vi "main.vi"() -> ()   [LabVIEW 2011]
uses:
  Controls/Full_90 Degree Pulse Settings.ctl
  Controls/90D_Delay Settings.ctl
  Controls/90D_Preliminary Settings.ctl
  Controls/90D_Pulse Settings.ctl
  Controls/Acquisition Settings.ctl
  Controls/Full_CPMG Degree Pulse Settings.ctl
  Controls/CPMG_Delay Settings.ctl
  Controls/CPMG_Preliminary Settings.ctl
  Controls/CPMG_Pulse Settings.ctl
  Controls/Full_T1 Degree Pulse Settings.ctl
  Controls/T1_Preliminary Settings.ctl
  Controls/T1_Pulse Settings.ctl
  Controls/T1_Delay Settings.ctl
  Controls/Hardware Control.ctl
  Controls/NMR Pulse Sequence Type.ctl
  Controls/Class Objects.ctl
  Modules/File/Configuration/Configuration.lvclass
  Modules/File/TDMS/TDMS.lvclass
  Modules/Hardware/Power Supply/Power Supply.lvclass
  Modules/Hardware/NMR/NMR.lvclass
  Controls/User Event Control.ctl
  Controls/User Event Action.ctl
  Controls/User Interface Control.ctl
  Controls/User Interface Action.ctl
  <vilib>/Utility/error.llb/DialogType.ctl
  Error Handling/Custom Errors.ctl
  Functional Globals/Pulse Parameters.ctl
  Error Handling/Error Module Action.ctl
  Functional Globals/General Flags.ctl
  Functional Globals/Hardware Parameters.ctl
  Controls/Class Labels.ctl
panel:
  in  "Tab Control":T1(tab)
  out "FFT Graph":cluster{"magnitude":dbl[], dbl[]}[](graph)
  out "Time Graph":cluster{"magnitude":dbl[], dbl[]}[](graph)
  in  "Hardware CTRL":T2={"Number Samples"=5000, "Time Between Points"=10.0, "Gain2 (dB)"=12, "CuttOff Freq1[MHz]"=10, "CuttOff Freq2[MHz]"=1, "Frequency"=10000000.0, "Phase"=180, "Power Level"=230, "Send Pulse"=FALSE, "Reset DDS"=FALSE, "TX CTRL"=FALSE, "RX CTRL"=TRUE, "Gain1 (dB)"=5, "Set DDS"=FALSE, "Start AQS"=FALSE, "Units"=0} {"Units" items=["us", "ms"]; "Gain1 (dB)" min=-5 max=45 step=1; "Power Level" max=1023 step=1; "Phase" max=270 step=90; "Frequency" min=1.0 format="%^#_6e"; "CuttOff Freq2[MHz]" min=1 max=30 step=1; "CuttOff Freq1[MHz]" min=1 max=30 step=1; "Gain2 (dB)" min=-5 max=45 step=1; "Time Between Points" min=0.0 step=1.0; "Number Samples" step=1}
  in  "Save to file":bool
  in  "Sum?":bool=TRUE
  out "Transfer Time (ms)":u32=322
  in  "start sequence  loop":bool
  out "Real (time Domain)":cluster{"magnitude":dbl[], dbl[]}(graph)
  out "Imag (Freq Domain)":cluster{"magnitude":dbl[], dbl[]}(graph)
  in  "Pulse Sequence Type":T3
  in  "90 Degree Pulse Sequence":T4={"Delay Settings"={"Delay d1"=99.98328812669524, "Delay d2"=3.0280548223167, "d1 Unit"=0, "d2 Unit"=1}, "Preliminary Settings"={"Nº of Scans (ns)"=20, "Pulse Frequency"=10000000.0}, "Pulse Settings"={"Duration Signal P1"=20.01128707673462, "Power Level"=800, "Phase"=90, "P1 Units"=0}, "Acquisition Settings"={"Number Samples"=8000, "Time Between Points"=0.0, "Unit"=0}} {"Acquisition Settings"."Unit" items=["us", "ms"]; "Acquisition Settings"."Time Between Points" min=0.0 step=1.0; "Acquisition Settings"."Number Samples" step=1; "Pulse Settings"."P1 Units" items=["us", "ms"]; "Pulse Settings"."Phase" max=270 step=90; "Pulse Settings"."Power Level" max=1023 step=1; "Pulse Settings"."Duration Signal P1" min=0.0 step=1.0 format="%#_4g"; "Preliminary Settings"."Pulse Frequency" min=1.0 max=200000000.0 step=1000000.0 format="%^#_6e"; "Preliminary Settings"."Nº of Scans (ns)" step=1; "Delay Settings"."d2 Unit" items=["us", "ms"]; "Delay Settings"."d1 Unit" items=["us", "ms"]; "Delay Settings"."Delay d2" min=0.0 step=1.0 format="%#_4g"; "Delay Settings"."Delay d1" min=0.0 step=1.0 format="%#_4g"}
  in  "start sequence":bool
  in  "CPMG Pulse Sequence":T9={"Acquisition Settings"={"Number Samples"=500, "Time Between Points"=20.0, "Unit"=0}, "Delay Settings"={"Delay d1"=100.0, "Delay d2"=2.0, "d1 Unit"=0, "d2 Unit"=0, "Delay d3"=100.0, "d3 Unit"=0, "Delay d4"=2.0, "d4 Unit"=0}, "Preliminary Settings"={"Nº of Scans (ns)"=2, "Pulse Frequency"=9000000.0, "Nº of Echoes (ne)"=3}, "Pulse Settings"={"Duration Signal P1"=100.0, "Power Level P1"=1000, "Phase P1"=90, "P1 Unit"=0, "Duration Signal P2"=100.0, "Power Level P2"=1000, "Phase P2"=90, "P2 Unit"=0}} {"Pulse Settings"."P2 Unit" items=["us", "ms"]; "Pulse Settings"."Phase P2" max=270 step=90; "Pulse Settings"."Power Level P2" max=1023 step=1; "Pulse Settings"."Duration Signal P2" min=0.0 step=1.0 format="%#_4g"; "Pulse Settings"."P1 Unit" items=["us", "ms"]; "Pulse Settings"."Phase P1" max=270 step=90; "Pulse Settings"."Power Level P1" max=1023 step=1; "Pulse Settings"."Duration Signal P1" min=0.0 step=1.0 format="%#_4g"; "Preliminary Settings"."Nº of Echoes (ne)" step=1; "Preliminary Settings"."Pulse Frequency" min=1.0 max=200000000.0 step=1000000.0 format="%^#_6e"; "Preliminary Settings"."Nº of Scans (ns)" step=1; "Delay Settings"."d4 Unit" items=["us", "ms"]; "Delay Settings"."Delay d4" min=0.0 step=1.0 format="%#_4g"; "Delay Settings"."d3 Unit" items=["us", "ms"]; "Delay Settings"."Delay d3" min=0.0 step=1.0 format="%#_4g"; "Delay Settings"."d2 Unit" items=["us", "ms"]; "Delay Settings"."d1 Unit" items=["us", "ms"]; "Delay Settings"."Delay d2" min=0.0 step=1.0 format="%#_4g"; "Delay Settings"."Delay d1" min=0.0 step=1.0 format="%#_4g"; "Acquisition Settings"."Unit" items=["us", "ms"]; "Acquisition Settings"."Time Between Points" min=0.0 step=1.0; "Acquisition Settings"."Number Samples" step=1}
  in  "T1 Pulse Sequence":T13={"Preliminary Settings"={"Nº of Scans (ns)"=2, "Pulse Frequency"=9000000.0, "Nº of Vd"=3}, "Pulse Settings"={"Duration Signal P2"=100.0, "Power Level P2"=1000, "Phase P2"=90, "P2 Unit"=0, "Duration Signal P1"=100.0, "Power Level P1"=1000, "Phase P1"=90, "P1 Unit"=0}, "Acquisition Settings"={"Number Samples"=5000, "Time Between Points"=20.0, "Unit"=0}, "Delay Settings"={"Delay d1"=100.0, "Delay d2"=2.0, "d1 Unit"=0, "d2 Unit"=0, "Delay d30"=0.0, "d30 Unit"=0, "Vd Unit"=0, "Vd Values"="Automatic"}} {"Delay Settings"."Vd Unit" items=["us", "ms"]; "Delay Settings"."d30 Unit" items=["us", "ms"]; "Delay Settings"."Delay d30" min=0.0 step=1.0; "Delay Settings"."d2 Unit" items=["us", "ms"]; "Delay Settings"."d1 Unit" items=["us", "ms"]; "Delay Settings"."Delay d2" min=0.0 step=1.0 format="%#_4g"; "Delay Settings"."Delay d1" min=0.0 step=1.0 format="%#_4g"; "Acquisition Settings"."Unit" items=["us", "ms"]; "Acquisition Settings"."Time Between Points" min=0.0 step=1.0; "Acquisition Settings"."Number Samples" step=1; "Pulse Settings"."P1 Unit" items=["us", "ms"]; "Pulse Settings"."Phase P1" max=270 step=90; "Pulse Settings"."Power Level P1" max=1023 step=1; "Pulse Settings"."Duration Signal P1" min=0.0 step=1.0 format="%#_4g"; "Pulse Settings"."P2 Unit" items=["us", "ms"]; "Pulse Settings"."Phase P2" max=270 step=90; "Pulse Settings"."Power Level P2" max=1023 step=1; "Pulse Settings"."Duration Signal P2" min=0.0 step=1.0 format="%#_4g"; "Preliminary Settings"."Nº of Vd" step=1; "Preliminary Settings"."Pulse Frequency" min=1.0 max=200000000.0 step=1000000.0 format="%^#_6e"; "Preliminary Settings"."Nº of Scans (ns)" step=1}
  out "Real (Freq Domain)":cluster{"magnitude":dbl[], dbl[]}(graph)
  out "Imag (time Domain)":cluster{"magnitude":dbl[], dbl[]}(graph)
  out "Sequence Progress":u32(slide)=20 scale=0.0..50.0
  out "Status Bar":string="Sequence Started"
  # "Sequence parameters:\n\nd30 - does not need to be configured"
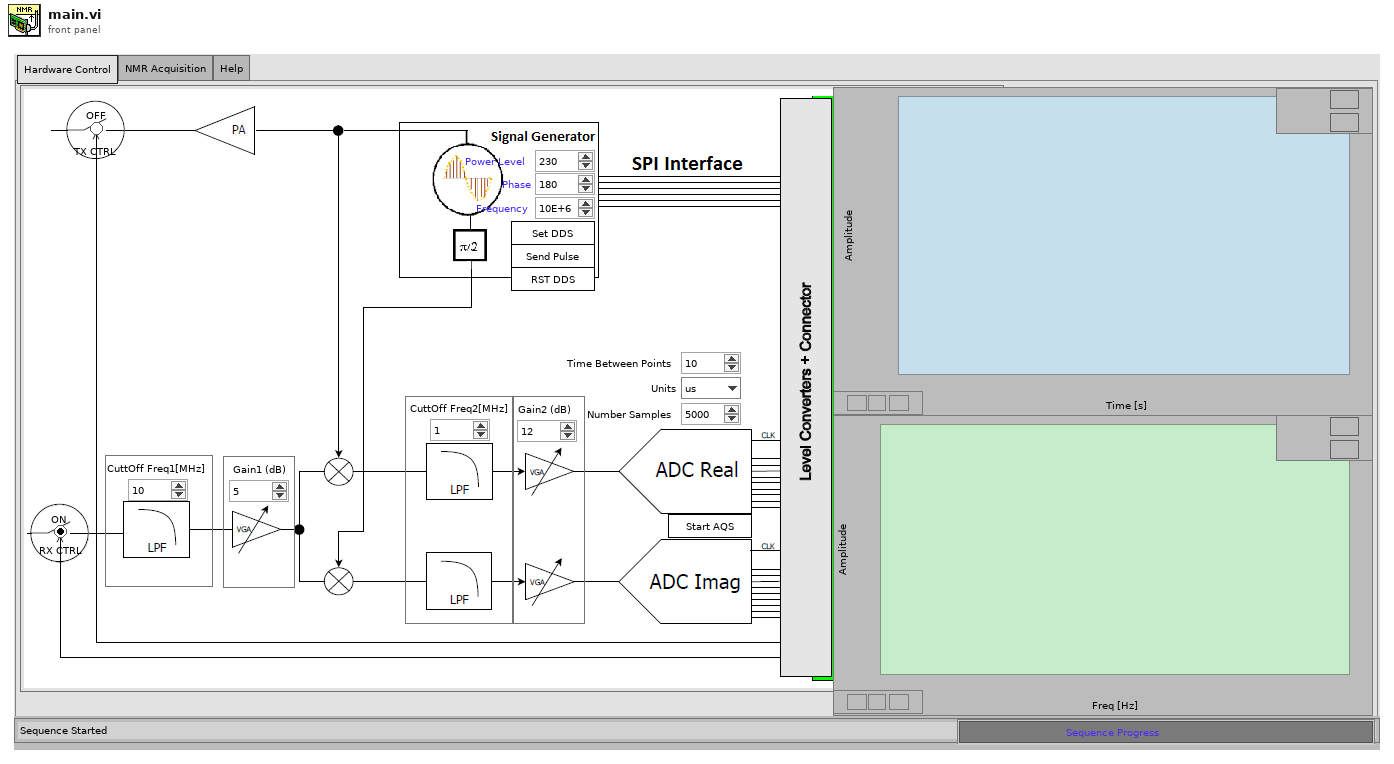
[diagram p1: front panel]
types:
  T1 = enum32{"Hardware Control", "NMR Acquisition", "Help"}
  T2 = typedef "Hardware Control.ctl" = cluster{"Number Samples":u16, "Time Between Points":dbl, "Gain2 (dB)":i8, "CuttOff Freq1[MHz]":u8, "CuttOff Freq2[MHz]":u8, "Frequency":dbl, "Phase":u16, "Power Level":u16, "Send Pulse":bool, "Reset DDS":bool, "TX CTRL":bool, "RX CTRL":bool, "Gain1 (dB)":i8, "Set DDS":bool, "Start AQS":bool, "Units":u8}
  T3 = typedef "NMR Pulse Sequence Type.ctl" = enum16{"90 Degree Sequence", "CPMG Pulse Sequence", "T1 Pulse Sequence"}
  T4 = typedef "Full_90 Degree Pulse Settings.ctl" = cluster{"Delay Settings":T5, "Preliminary Settings":T6, "Pulse Settings":T7, "Acquisition Settings":T8}
  T5 = typedef "90D_Delay Settings.ctl" = cluster{"Delay d1":dbl, "Delay d2":dbl, "d1 Unit":u8, "d2 Unit":u8}
  T6 = typedef "90D_Preliminary Settings.ctl" = cluster{"Nº of Scans (ns)":u16, "Pulse Frequency":dbl}
  T7 = typedef "90D_Pulse Settings.ctl" = cluster{"Duration Signal P1":dbl, "Power Level":u16, "Phase":u16, "P1 Units":u8}
  T8 = typedef "Acquisition Settings.ctl" = cluster{"Number Samples":u16, "Time Between Points":dbl, "Unit":u8}
  T9 = typedef "Full_CPMG Degree Pulse Settings.ctl" = cluster{"Acquisition Settings":T8, "Delay Settings":T10, "Preliminary Settings":T11, "Pulse Settings":T12}
  T10 = typedef "CPMG_Delay Settings.ctl" = cluster{"Delay d1":dbl, "Delay d2":dbl, "d1 Unit":u8, "d2 Unit":u8, "Delay d3":dbl, "d3 Unit":u8, "Delay d4":dbl, "d4 Unit":u8}
  T11 = typedef "CPMG_Preliminary Settings.ctl" = cluster{"Nº of Scans (ns)":u16, "Pulse Frequency":dbl, "Nº of Echoes (ne)":u16}
  T12 = typedef "CPMG_Pulse Settings.ctl" = cluster{"Duration Signal P1":dbl, "Power Level P1":u16, "Phase P1":u16, "P1 Unit":u8, "Duration Signal P2":dbl, "Power Level P2":u16, "Phase P2":u16, "P2 Unit":u8}
  T13 = typedef "Full_T1 Degree Pulse Settings.ctl" = cluster{"Preliminary Settings":T14, "Pulse Settings":T15, "Acquisition Settings":T8, "Delay Settings":T16}
  T14 = typedef "T1_Preliminary Settings.ctl" = cluster{"Nº of Scans (ns)":u16, "Pulse Frequency":dbl, "Nº of Vd":u16}
  T15 = typedef "T1_Pulse Settings.ctl" = cluster{"Duration Signal P2":dbl, "Power Level P2":u16, "Phase P2":u16, "P2 Unit":u8, "Duration Signal P1":dbl, "Power Level P1":u16, "Phase P1":u16, "P1 Unit":u8}
  T16 = typedef "T1_Delay Settings.ctl" = cluster{"Delay d1":dbl, "Delay d2":dbl, "d1 Unit":u8, "d2 Unit":u8, "Delay d30":dbl, "d30 Unit":u8, "Vd Unit":u8, "Vd Values":string}
  T17 = typedef "User Interface Control.ctl" = cluster{"data1":variant, "data2":variant, "action":T18}
  T18 = typedef "User Interface Action.ctl" = enum16{"Initialize", "Update Real Channel", "Update Imag Channel", "Update Re/Im channel @ Hardware Ctrl", "Pulse Sequence", "Visibility Front Panel Controls", "Report Custom Errors", "Set Pulse Sequence Type", "Update Pulse Timings", "Update Transfer Time", "Update Status Bar", "Set Sequence Progress", "Set 90 Degree Pulse Sequence Params", "Set CMPG Pulse Sequence Parms", "Set T1 Pulse Sequence Params", "Stop"}
  T19 = typedef "User Event Control.ctl" = cluster{"data":variant, "action":T20}
  T20 = typedef "User Event Action.ctl" = enum16{"Initialize", "Shutdown", "Start NMR DAQ", "Start NMR DAQ Loop", "Set DDS", "Reset DDS", "Send Pulse", "Set TX SW", "Set RX SW", "Set CutOff Freq1", "Set CutOff Freq2", "Set Gain1", "Set Gain2", "Start AQS", "Configure Device Settings"}
  T21 = typedef "Class Objects.ctl" = cluster{"configuration":refnum<class "Configuration.lvclass">, "TDMS":refnum<class "TDMS.lvclass">[], "Power Supply":refnum<class "Power Supply.lvclass">, "NMR":refnum<class "NMR.lvclass">}
  T22 = typedef "Hardware Parameters.ctl" = enum16{"Initialize", "Set Hardware Settings", "Get Hardware Settings", "Get Hardware CMD String"}
  T23 = typedef "Pulse Parameters.ctl" = enum16{"Initialize", "Set T1 Pulse Settings", "Set 90 Degree Pulse Settings", "Set CPMG Pulse Settings", "Get T1 Settings", "Get CPMG Settings", "Get 90 Degree Settings"}
  T24 = typedef "Class Labels.ctl" = enum16{"Configuration", "TDMS", "Detector", "Power Supply", "MFC", "NMR", "Valve Controller"}
  T25 = cluster{"Delay Settings":T5, "Preliminary Settings":T6, "Pulse Settings":T7, "Acquisition Settings":T8}
  T26 = cluster{"Acquisition Settings":T8, "Delay Settings":T10, "Preliminary Settings":T11, "Pulse Settings":T12}
  T27 = cluster{"Preliminary Settings":T14, "Pulse Settings":T15, "Acquisition Settings":T8, "Delay Settings":T16}
  T28 = typedef "Error Module Action.ctl" = enum16{"Initialize", "Handle Errors", "Report Errors"}
  T29 = typedef "General Flags.ctl" = enum16{"Initialize", "Set Abort Flag", "Get Abort Flag"}
  T30 = cluster{"Number Samples":u16, "Time Between Points":dbl, "Gain2 (dB)":i8, "CuttOff Freq1[MHz]":u8, "CuttOff Freq2[MHz]":u8, "Frequency":dbl, "Phase":u16, "Power Level":u16, "Send Pulse":bool, "Reset DDS":bool, "TX CTRL":bool, "RX CTRL":bool, "Gain1 (dB)":i8, "Set DDS":bool, "Start AQS":bool, "Units":u8}
  T31 = typedef "Custom Errors.ctl" = cluster{"[user-defined codes]":i32[], "[user-defined descriptions]":string[]}
  T32 = typedef "DialogType.ctl" = u16
  T33 = cluster{"D1 Real Time":ext, "D2 Real Time":ext, "P1 Real Time":ext, "AQS Real Time":ext}
  T34 = cluster{"Real Time d4":ext, "Real Time d3":ext, "Real Time P2":ext, "Real Time d2":ext, "Real Time P1":ext, "Real Time d1":ext, "Real Time AQS":ext}
  T35 = cluster{"Real Time P1":ext, "Real Time P2":ext, "Real Time d1":ext, "Real Time d2":ext, "Real Time d30":ext, "Real Time AQS":ext}
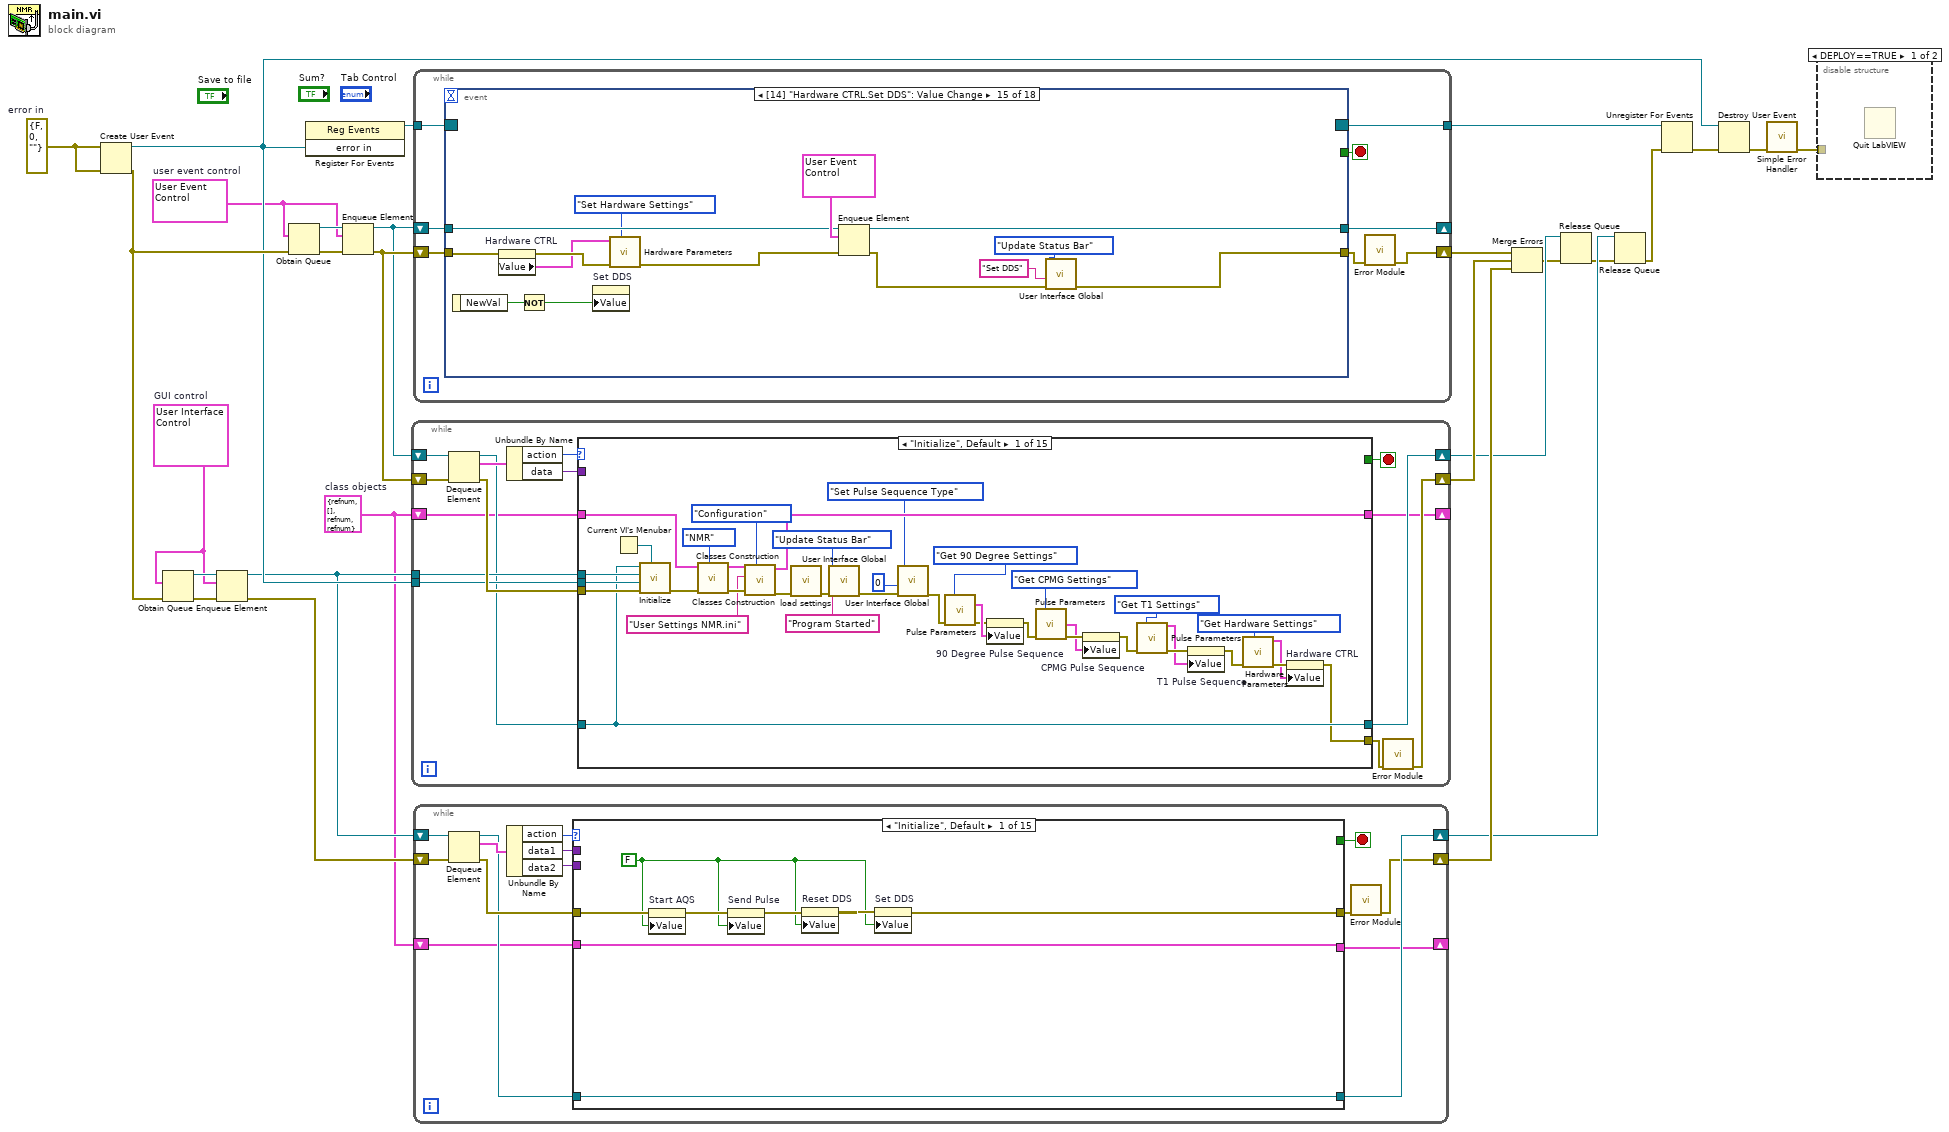
[diagram p0: block diagram]
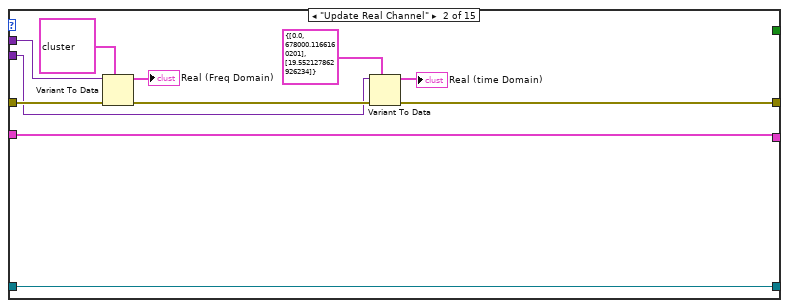
[diagram p3: hidden frame]
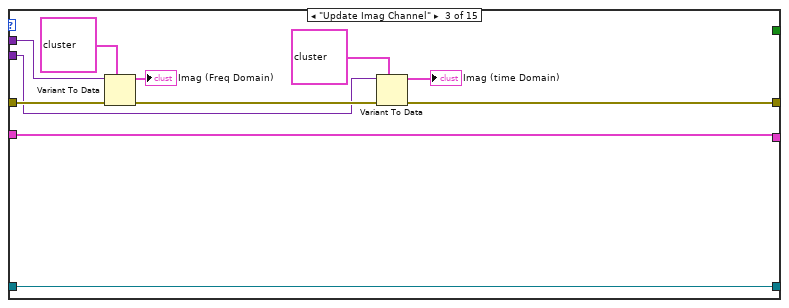
[diagram p4: hidden frame]
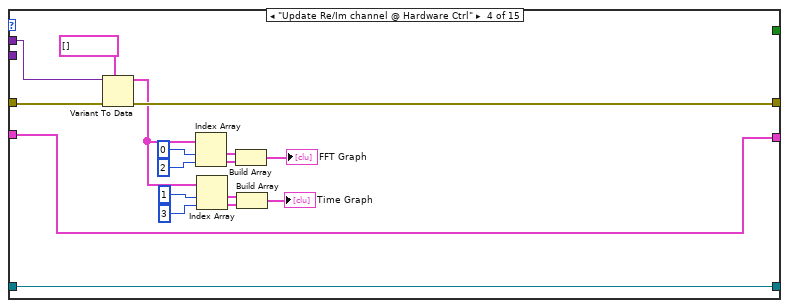
[diagram p5: hidden frame]
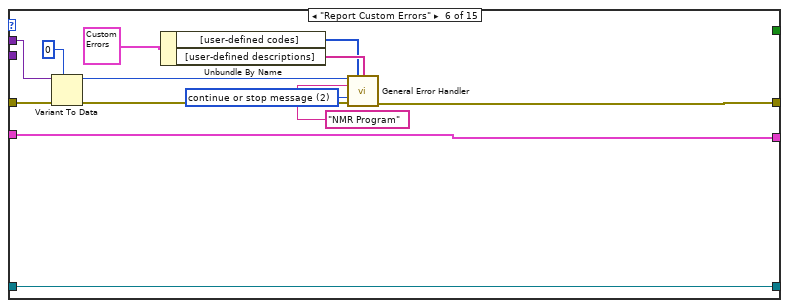
[diagram p7: hidden frame]
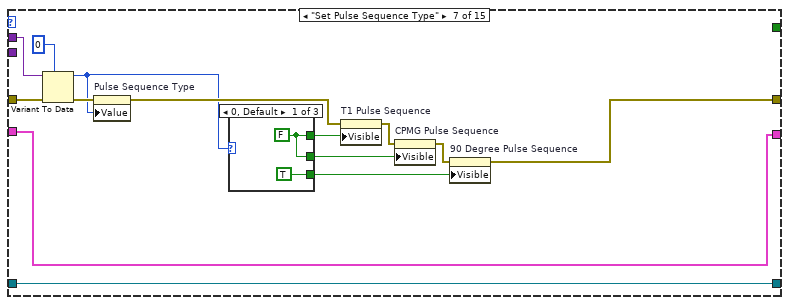
[diagram p8: hidden frame]
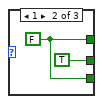
[diagram p9: hidden frame]
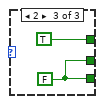
[diagram p10: hidden frame]
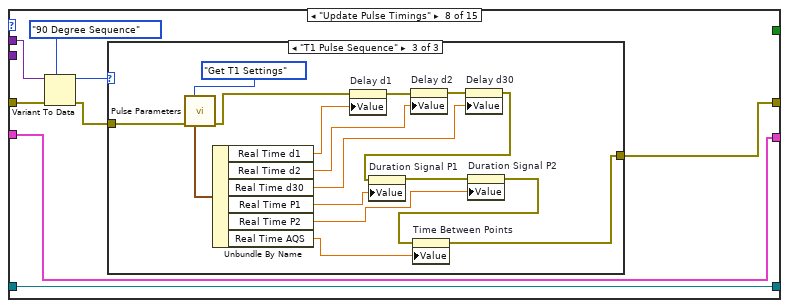
[diagram p11: hidden frame]
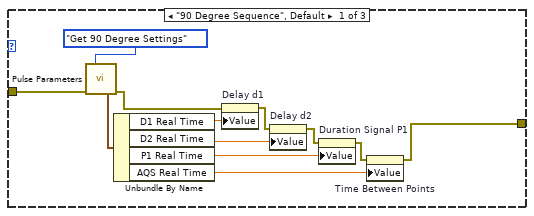
[diagram p12: hidden frame]
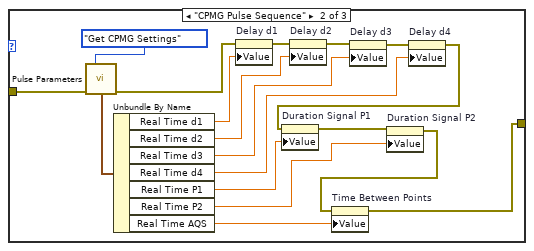
[diagram p13: hidden frame]
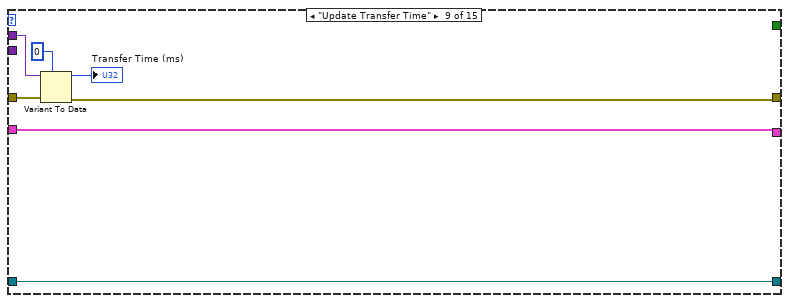
[diagram p14: hidden frame]
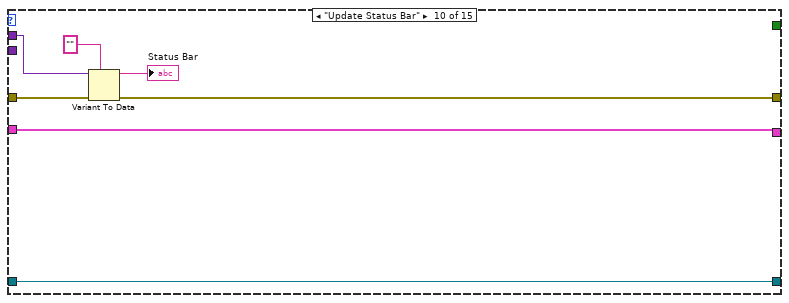
[diagram p15: hidden frame]
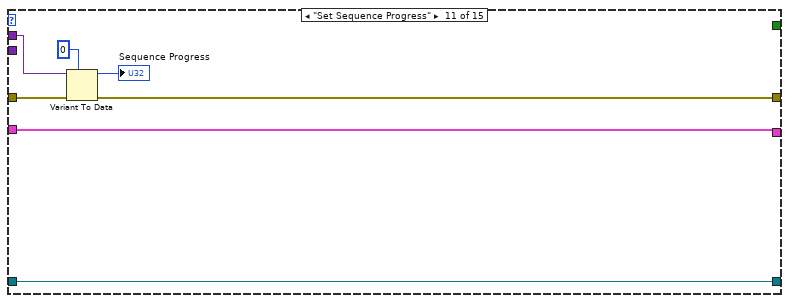
[diagram p16: hidden frame]
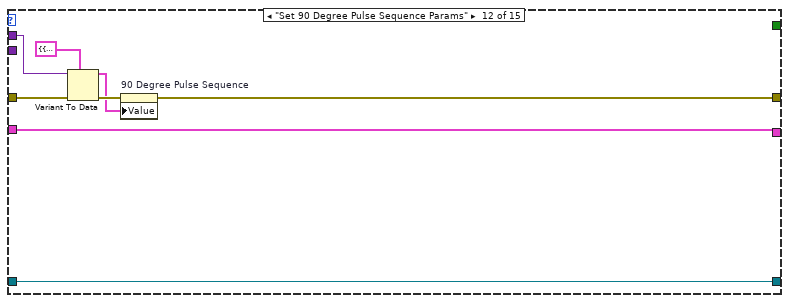
[diagram p17: hidden frame]
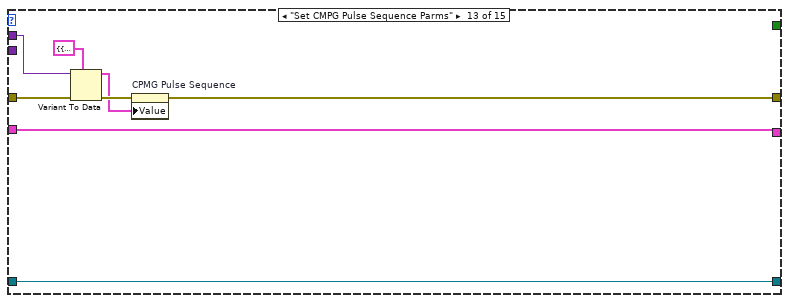
[diagram p18: hidden frame]
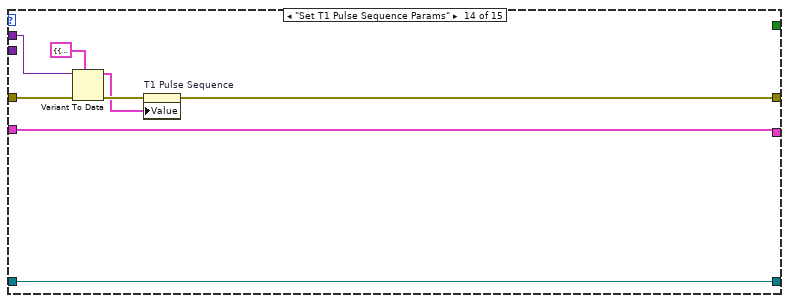
[diagram p19: hidden frame]
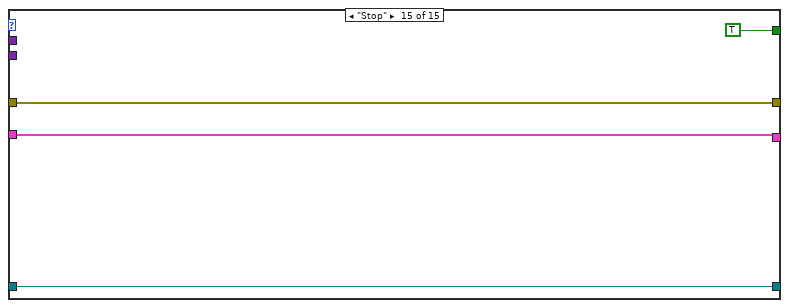
[diagram p20: hidden frame]
diagram:
  w3 = T17 {"data1"=variant, "data2"=variant, "action"=enum."Initialize"}  # GUI control
  w4 = T19 {"data"=variant, "action"=enum."Initialize"}  # user event control
  w1 = T21 {"configuration"=refnum, "TDMS"=[], "Power Supply"=refnum, "NMR"=refnum}  # class objects
  w6 = errorcluster {"status"=FALSE, "code"=0, "source"=""}  # error in
  n1 = Create User Event(user event datatype=w6, error in=w6) -> (user event=w7:refnum<user-event>, error out=w21:errorcluster)
  n2 = Obtain Queue(element data type=w3, error in (no error)=w21) -> (queue out=w22:refnum<queue>, error out=w23:errorcluster)  [unwired: 3 in, 1 out]
  n3 = Enqueue Element(queue=w22, element=w3, error in (no error)=w23) -> (queue out=w5:refnum<queue>, error out=w20:errorcluster)  [unwired: 1 in, 1 out]
  n4 = Obtain Queue(element data type=w4, error in (no error)=w21) -> (queue out=w24:refnum<queue>, error out=w25:errorcluster)  [unwired: 3 in, 1 out]
  n5 = register-events(w7) -> (reference out=w27:refnum<event-registration>)  [unwired: 2 in, 1 out]
  n6 = Enqueue Element(queue=w24, element=w4, error in (no error)=w25) -> (queue out=w8:refnum<queue>, error out=w19:errorcluster)  [unwired: 1 in, 1 out]
  n7 = while {
    shift-right: [w36] -> w15
    shift-left: w8 -> [w42]
    shift-right: [w34] -> w17
    shift-left: w19 -> [w41]
    tunnel: w5 -> [w33]
    tunnel: w7 -> [w32]
    shift-right: [w28] -> _
    shift-left: w1 -> [w30]
    stop <- w35 stop-if-true
    n8 = Dequeue Element(queue=w42, error in (no error)=w41) -> (queue out=w31:refnum<queue>, element=w40:T19, error out=w37:errorcluster)  [unwired: 1 in, 1 out]
    n9 = Unbundle By Name(w40) -> ("action"=w39:T20, "data"=w38:variant)
    n10 = case shown="\"Initialize\", Default" w39 {
      tunnel: w38 -> [_ _ _ _ _ _ _ _ _ _ _ _ _ _ _]
      tunnel: w37 -> [w79 w90 w110 w130 w142 w151 w164 w176 w188 w199 w210 w221 w232 w243 w251]
      tunnel: w31 -> [w75 w92 w114 w136 w149 w158 w171 w183 w195 w206 w217 w228 w239 w247 w249]
      tunnel: [w75 w92 w114 w136 w149 w158 w171 w183 w195 w206 w217 w228 w239 w247 w249] -> w36
      tunnel: [w43 w83 w106 w134 w145 w154 w167 w179 w191 w202 w213 w224 w235 w240 w250] -> w29
      tunnel: [_ TRUE _ _ _ _ _ _ _ _ _ _ _ _ _] -> w35
      tunnel: w33 -> [w76 w89 _ _ _ _ _ _ _ _ _ _ _ _ _]
      tunnel: w32 -> [w78 _ _ _ _ _ _ _ _ _ _ _ _ _ _]
      tunnel: w30 -> [w72 w88 w109 w132 w147 w156 w169 w181 w193 w204 w215 w226 w237 w246 w248]
      tunnel: [w69 w84 w113 w131 w144 w153 w166 w178 w190 w201 w212 w223 w234 w245 w248] -> w28
      frame "Initialize", Default {
        n11 = Current VI's Menubar() -> (w77:refnum<k9>)
        n12 = call "Initialize.vi"("menu ref"=w77, "error in"=w79, "dynamic event queue reference"=w78, "User Interface Control Reference"=w76, "User Event Control Reference"=w75) -> ("error out"=w74:errorcluster)  [unwired: 6 in]
        n13 = call "Classes Construction.vi"("class"=Class_Labels."NMR", "error in"=w74, "objects"=w72) -> ("error out"=w70:errorcluster, "objects"=w71:T21)  [unwired: 5 in, 1 out]
        n14 = call "Classes Construction.vi"("class"=Class_Labels."Configuration", "error in"=w70, "param1"="User Settings NMR.ini", "objects"=w71) -> ("error out"=w60:errorcluster, "objects"=w69:T21)  [unwired: 4 in, 1 out]
        n15 = call "load settings.vi"("error in (no error)"=w60) -> ("error out"=w59:errorcluster)  [unwired: 9 in, 1 out]
        n16 = call "User Interface Global.vi"("error in"=w59, "data1"="Program Started", "action"=User_Interface_Action."Update Status Bar") -> ("error out"=w64:errorcluster)  [unwired: 8 in]
        n17 = call "User Interface Global.vi"("error in"=w64, "data1"=0, "action"=User_Interface_Action."Set Pulse Sequence Type") -> ("error out"=w63:errorcluster)  [unwired: 8 in]
        n18 = call "Pulse Parameters.vi"("action"=Pulse_Parameters."Get 90 Degree Settings", "error in"=w63) -> ("90 Degree Pulse settings out"=w55:T25, "error out"=w54:errorcluster)  [unwired: 6 in, 6 out]
        n19 = property on="90 Degree Pulse Sequence" class="Clust (strict)"(error in=w54, "Value"=w55) -> (error out=w53:errorcluster)  [unwired: 1 in, 1 out]
        n20 = call "Pulse Parameters.vi"("action"=Pulse_Parameters."Get CPMG Settings", "error in"=w53) -> ("CPMG pulse settings Out"=w51:T26, "error out"=w52:errorcluster)  [unwired: 6 in, 6 out]
        n21 = property on="CPMG Pulse Sequence" class="Clust (strict)"(error in=w52, "Value"=w51) -> (error out=w50:errorcluster)  [unwired: 1 in, 1 out]
        n22 = call "Pulse Parameters.vi"("action"=Pulse_Parameters."Get T1 Settings", "error in"=w50) -> ("T1 Pulse settings Out"=w48:T27, "error out"=w49:errorcluster)  [unwired: 6 in, 6 out]
        n23 = property on="T1 Pulse Sequence" class="Clust (strict)"(error in=w49, "Value"=w48) -> (error out=w47:errorcluster)  [unwired: 1 in, 1 out]
        n24 = call "Hardware Parameters.vi"("action"=Hardware_Parameters."Get Hardware Settings", "error in"=w47) -> ("error out"=w45:errorcluster, "Hardware Paramentes out"=w44:T2)  [unwired: 8 in]
        n25 = property on="Hardware CTRL" class="Clust (strict)"(error in=w45, "Value"=w44) -> (error out=w43:errorcluster)  [unwired: 1 in, 1 out]
      }
      frame "Shutdown" {
        n26 = call "Shutdown.vi"("error in"=w90, "User Interface Control Reference"=w89) -> ("error out"=w81:errorcluster)  [unwired: 9 in]
        n27 = call "save_settings.vi"("error in"=w81) -> ("error out"=w80:errorcluster)  [unwired: 9 in, 1 out]
        n28 = call "Classes Destruction.vi"("class labels"=Class_Labels."NMR", "error in"=w80, "objects"=w88) -> ("error out"=w85:errorcluster, "objects"=w86:T21)  [unwired: 7 in]
        n29 = call "Classes Destruction.vi"("class labels"=Class_Labels."Configuration", "error in"=w85, "objects"=w86) -> ("error out"=w83:errorcluster, "objects"=w84:T21)  [unwired: 7 in]
      }
      frame "Start NMR DAQ" {
        n30 = First Call?() -> (First Call?: T/F=w107:bool)
        n31 = case shown="True" w107 {
          tunnel: w110 -> [w115 w121]
          tunnel: [w115 w119] -> w101
          tunnel: w109 -> [w116 w118]
          tunnel: [w116 w117] -> w108
          frame False {
          }
          frame True {
            n32 = call "Classes Construction.vi"("class"=Class_Labels."TDMS", "error in"=w121, "objects"=w118) -> ("error out"=w119:errorcluster, "objects"=w117:T21)  [unwired: 5 in, 1 out]
          }
        }
        n33 = property on="start sequence  loop" class="Bool (strict)"(error in=w101, "Visible"=FALSE) -> (error out=w95:errorcluster)  [unwired: 1 in, 1 out]
        n34 = call "User Interface Global.vi"("error in"=w95, "data1"="Sequence Started", "action"=User_Interface_Action."Update Status Bar") -> ("error out"=w94:errorcluster)  [unwired: 8 in]
        n35 = control-ref of="Sequence Progress"() -> (w104:refnum<vi>)
        n36 = local read "Save to file"() -> (w93:bool)
        n37 = property on="Pulse Sequence Type" class="Enum (strict)"(error in=w94) -> (error out=w111:errorcluster, "Value"=w112:T3)  [unwired: 1 in, 1 out]
        n38 = local read "Sum?"() -> (w103:bool)
        n39 = call "Execute Sequence.vi"("Sequence Progress"=w104, "Pulse Sequence Type"=w112, "Sum?"=w103, "error in (no error)"=w111, "Save File"=w93, "class objects in"=w108) -> ("error out"=w99:errorcluster, "class objects out"=w113:T21)  [unwired: 2 in, 2 out]
        n40 = property on="start sequence  loop" class="Bool (strict)"(error in=w99, "Visible"=TRUE) -> (error out=w98:errorcluster)  [unwired: 1 in, 1 out]
        n41 = property on="start sequence" class="Bool (strict)"(error in=w98, "Value"=FALSE ("start sequence")) -> (error out=w106:errorcluster)  [unwired: 1 in, 1 out]
      }
      frame "Start NMR DAQ Loop" {
        n42 = property on="start sequence" class="Bool (strict)"(error in=w130, "Visible"=FALSE) -> (error out=w129:errorcluster)  [unwired: 1 in, 1 out]
        n43 = control-ref of="Sequence Progress"() -> (w135:refnum<vi>)
        n44 = call "Execute Sequence Loop.vi"("Sequence Progress"=w135, "error in (no error)"=w129, "class objects in"=w132) -> ("error out"=w126:errorcluster, "class objects Out"=w131:T21)  [unwired: 7 in]
        n45 = property on="start sequence" class="Bool (strict)"(error in=w126, "Visible"=TRUE) -> (error out=w123:errorcluster)  [unwired: 1 in, 1 out]
        n46 = call "User Interface Global.vi"("error in"=w123, "data1"="Sequence Loop Started - 100% Done", "action"=User_Interface_Action."Update Status Bar") -> ("error out"=w124:errorcluster)  [unwired: 8 in]
        n47 = property on="start sequence  loop" class="Bool (strict)"(error in=w124, "Value"=FALSE ("start sequence  loop")) -> (error out=w134:errorcluster)  [unwired: 1 in, 1 out]
      }
      frame "Set DDS" {
        n48 = call "Hardware Parameters.vi"("action"=Hardware_Parameters."Get Hardware Settings", "error in"=w142) -> ("error out"=w141:errorcluster, "Hardware Paramentes out"=w140:T2)  [unwired: 8 in]
        n49 = Unbundle By Name(w140) -> ("Power Level"=w139:u16, "Phase"=w138:u16, "Frequency"=w137:dbl)
        n50 = Unbundle By Name(w147) -> ("NMR"=w148:refnum<class "NMR.lvclass">)
        n51 = call-dynamic "Set DDS.vi"("NMR in"=w148, "Power Level"=w139, "Phase"=w138, "Frequency"=w137, "error in (no error)"=w141) -> ("NMR out"=w146:refnum<class "NMR.lvclass">, "error out"=w145:errorcluster)  [unwired: 8 in, 1 out]
        n52 = Bundle By Name(cluster=w147, "NMR"=w146) -> (w144:T21)
      }
      frame "Reset DDS" {
        n53 = call "Hardware Parameters.vi"("action"=Hardware_Parameters."Get Hardware Settings", "error in"=w151) -> ("error out"=w150:errorcluster)  [unwired: 8 in, 1 out]
        n54 = Unbundle By Name(w156) -> ("NMR"=w157:refnum<class "NMR.lvclass">)
        n55 = call-dynamic "Reset DDS.vi"("error in (no error)"=w150, "NMR in"=w157) -> ("error out"=w154:errorcluster, "NMR out"=w155:refnum<class "NMR.lvclass">)  [unwired: 7 in, 1 out]
        n56 = Bundle By Name(cluster=w156, "NMR"=w155) -> (w153:T21)
      }
      frame "Send Pulse" {
        n57 = call "Hardware Parameters.vi"("action"=Hardware_Parameters."Get Hardware Settings", "error in"=w164) -> ("error out"=w163:errorcluster, "Hardware Paramentes out"=w162:T2)  [unwired: 8 in]
        n58 = Unbundle By Name(w162) -> ("Power Level"=w161:u16, "Phase"=w160:u16, "Frequency"=w159:dbl)
        n59 = Unbundle By Name(w169) -> ("NMR"=w170:refnum<class "NMR.lvclass">)
        n60 = call-dynamic "SendPulse DDS.vi"("NMR in"=w170, "Power Level"=w161, "Phase"=w160, "Frequency"=w159, "error in (no error)"=w163) -> ("NMR out"=w168:refnum<class "NMR.lvclass">, "error out"=w167:errorcluster)  [unwired: 8 in, 1 out]
        n61 = Bundle By Name(cluster=w169, "NMR"=w168) -> (w166:T21)
      }
      frame "Set TX SW" {
        n62 = call "Hardware Parameters.vi"("action"=Hardware_Parameters."Get Hardware Settings", "error in"=w176) -> ("error out"=w175:errorcluster, "Hardware Paramentes out"=w174:T2)  [unwired: 8 in]
        n63 = Unbundle By Name(w174) -> ("TX CTRL"=w173:bool)
        n64 = Unbundle By Name(w181) -> ("NMR"=w182:refnum<class "NMR.lvclass">)
        n65 = Not(x=w173) -> (.not. x?=w172:bool)
        n66 = call-dynamic "Set TX SW.vi"("NMR in"=w182, "On/Off"=w172, "error in (no error)"=w175) -> ("NMR out"=w180:refnum<class "NMR.lvclass">, "error out"=w179:errorcluster)  [unwired: 10 in, 1 out]
        n67 = Bundle By Name(cluster=w181, "NMR"=w180) -> (w178:T21)
      }
      frame "Set RX SW" {
        n68 = call "Hardware Parameters.vi"("action"=Hardware_Parameters."Get Hardware Settings", "error in"=w188) -> ("error out"=w187:errorcluster, "Hardware Paramentes out"=w186:T2)  [unwired: 8 in]
        n69 = Unbundle By Name(w186) -> ("RX CTRL"=w185:bool)
        n70 = Unbundle By Name(w193) -> ("NMR"=w194:refnum<class "NMR.lvclass">)
        n71 = Not(x=w185) -> (.not. x?=w184:bool)
        n72 = call-dynamic "Set RX SW.vi"("NMR in"=w194, "On/Off"=w184, "error in (no error)"=w187) -> ("NMR out"=w192:refnum<class "NMR.lvclass">, "error out"=w191:errorcluster)  [unwired: 10 in, 1 out]
        n73 = Bundle By Name(cluster=w193, "NMR"=w192) -> (w190:T21)
      }
      frame "Set CutOff Freq1" {
        n74 = call "Hardware Parameters.vi"("action"=Hardware_Parameters."Get Hardware Settings", "error in"=w199) -> ("error out"=w198:errorcluster, "Hardware Paramentes out"=w197:T2)  [unwired: 8 in]
        n75 = Unbundle By Name(w197) -> ("CuttOff Freq1[MHz]"=w196:u8)
        n76 = Unbundle By Name(w204) -> ("NMR"=w205:refnum<class "NMR.lvclass">)
        n77 = call-dynamic "SET LPF1.vi"("NMR in"=w205, "CuttOff Freq [MHz]"=w196, "error in (no error)"=w198) -> ("NMR out"=w203:refnum<class "NMR.lvclass">, "error out"=w202:errorcluster)  [unwired: 10 in, 1 out]
        n78 = Bundle By Name(cluster=w204, "NMR"=w203) -> (w201:T21)
      }
      frame "Set CutOff Freq2" {
        n79 = call "Hardware Parameters.vi"("action"=Hardware_Parameters."Get Hardware Settings", "error in"=w210) -> ("error out"=w209:errorcluster, "Hardware Paramentes out"=w208:T2)  [unwired: 8 in]
        n80 = Unbundle By Name(w208) -> ("CuttOff Freq2[MHz]"=w207:u8)
        n81 = Unbundle By Name(w215) -> ("NMR"=w216:refnum<class "NMR.lvclass">)
        n82 = call-dynamic "SET LPF2.vi"("NMR in"=w216, "CuttOff Freq [MHz]"=w207, "error in (no error)"=w209) -> ("NMR out"=w214:refnum<class "NMR.lvclass">, "error out"=w213:errorcluster)  [unwired: 10 in, 1 out]
        n83 = Bundle By Name(cluster=w215, "NMR"=w214) -> (w212:T21)
      }
      frame "Set Gain1" {
        n84 = call "Hardware Parameters.vi"("action"=Hardware_Parameters."Get Hardware Settings", "error in"=w221) -> ("error out"=w220:errorcluster, "Hardware Paramentes out"=w219:T2)  [unwired: 8 in]
        n85 = Unbundle By Name(w219) -> ("Gain1 (dB)"=w218:i8)
        n86 = Unbundle By Name(w226) -> ("NMR"=w227:refnum<class "NMR.lvclass">)
        n87 = call-dynamic "Set Gain1.vi"("NMR in"=w227, "Gain (dB)"=w218, "error in (no error)"=w220) -> ("NMR out"=w225:refnum<class "NMR.lvclass">, "error out"=w224:errorcluster)  [unwired: 10 in, 1 out]
        n88 = Bundle By Name(cluster=w226, "NMR"=w225) -> (w223:T21)
      }
      frame "Set Gain2" {
        n89 = call "Hardware Parameters.vi"("action"=Hardware_Parameters."Get Hardware Settings", "error in"=w232) -> ("error out"=w231:errorcluster, "Hardware Paramentes out"=w230:T2)  [unwired: 8 in]
        n90 = Unbundle By Name(w230) -> ("Gain2 (dB)"=w229:i8)
        n91 = Unbundle By Name(w237) -> ("NMR"=w238:refnum<class "NMR.lvclass">)
        n92 = call-dynamic "Set Gain2.vi"("NMR in"=w238, "Gain (dB)"=w229, "error in (no error)"=w231) -> ("NMR out"=w236:refnum<class "NMR.lvclass">, "error out"=w235:errorcluster)  [unwired: 10 in, 1 out]
        n93 = Bundle By Name(cluster=w237, "NMR"=w236) -> (w234:T21)
      }
      frame "Start AQS" {
        n94 = call "Hardware Parameters.vi"("action"=Hardware_Parameters."Get Hardware Settings", "error in"=w243) -> ("error out"=w242:errorcluster, "Hardware Paramentes out"=w241:T2)  [unwired: 8 in]
        n95 = call "Hardware Aquisition.vi"("error in (no error)"=w242, "Hardware Paramentes In"=w241, "class objects in"=w246) -> ("error out"=w240:errorcluster, "class objects out"=w245:T21)  [unwired: 7 in]
      }
      frame "Configure Device Settings" {
        n96 = call "Device  settings.vi"("error in"=w251) -> ("error out"=w250:errorcluster)  [unwired: 10 in]
      }
    }
    n97 = call "Error Module.vi"("error in"=w29) -> ("error out"=w34:errorcluster)  [unwired: 9 in, 1 out]
  }
  n98 = while {
    tunnel: w27 -> [w259]
    tunnel: [w258] -> w26
    shift-right: [w253] -> _
    shift-left: w8 -> [w256]
    shift-right: [w254] -> w18
    shift-left: w19 -> [w257]
    stop <- w252 stop-if-true
    n99 = event shown="[14] \"Hardware CTRL.Set DDS\": Value Change" {
      selector: w259 -> [_ _ _ _ _ _ _ _ _ _ _ _ _ _ _ _ _ _]
      dyn-events: [_ _ _ _ _ _ _ _ _ _ _ _ _ _ _ _ _ _] -> w258
      timeout: _ -> [_ _ _ _ _ _ _ _ _ _ _ _ _ _ _ _ _ _]
      tunnel: w257 -> [w264 w283 w293 w298 w319 w341 w367 w373 w387 w404 w421 w435 w447 w459 w473 w487 w499 w510]
      tunnel: [w261 w281 w289 w295 w317 w349 w364 w369 w383 w400 w417 w431 w443 w455 w469 w483 w495 w507] -> w255
      tunnel: w256 -> [w263 w284 w291 w297 w320 w355 w366 w378 w398 w415 w429 w441 w453 w467 w481 w493 w505 w509]
      tunnel: [w262 w284 w291 w296 w318 w355 w366 w377 w397 w414 w428 w440 w452 w466 w480 w492 w502 w509] -> w253
      tunnel: [w260 TRUE _ _ _ _ _ _ _ _ _ _ _ _ _ _ _ _] -> w252
      event Menu Selection (User) {
        n100 = event-data() -> ("ItemTag"=w265:string)  [unwired: 1 in]
        n101 = case shown="\"Exit\", Default" w265 {
          tunnel: w264 -> [w267 w271 w279]
          tunnel: w263 -> [w268 w272 w278]
          tunnel: [w268 w270 w277] -> w262
          tunnel: [w266 w269 w276] -> w261
          tunnel: [_ _ TRUE] -> w260
          frame "About" {
            n102 = call "About_INL.vi"("error in"=w267) -> ("error out"=w266:errorcluster)  [unwired: 10 in]
          }
          frame "Device Settings" {
            n103 = Enqueue Element(queue=w272, element=T19 {"data"=variant, "action"=enum."Configure Device Settings"}, error in (no error)=w271) -> (queue out=w270:refnum<queue>, error out=w269:errorcluster)  [unwired: 1 in, 1 out]
          }
          frame "Exit", Default {
            n104 = Enqueue Element(queue=w278, element=T19 {"data"=variant, "action"=enum."Shutdown"} ("user event control"), error in (no error)=w279) -> (queue out=w277:refnum<queue>, error out=w276:errorcluster)  [unwired: 1 in, 1 out]
          }
        }
      }
      event User Event {
        n105 = event-data() -> ()  [unwired: 1 in, 1 out]
        n106 = call "Error Module.vi"("command (handle errors)"=Error_Module_Action."Report Errors", "error in"=w283) -> ("error out"=w281:errorcluster)  [unwired: 8 in, 1 out]
      }
      event Value Change {
        n107 = event-data() -> ("NewVal"=w285:T4)  [unwired: 1 in]
        n108 = call "Pulse Parameters.vi"("action"=Pulse_Parameters."Set 90 Degree Pulse Settings", "90 Degree Pulse Sequence"=w285, "error in"=w293) -> ("error out"=w288:errorcluster)  [unwired: 5 in, 7 out]
        n109 = property on="Pulse Sequence Type" class="Enum (strict)"(error in=w288) -> (error out=w287:errorcluster, "Value"=w286:T3)  [unwired: 1 in, 1 out]
        n110 = call "User Interface Global.vi"("error in"=w287, "data1"=w286, "action"=User_Interface_Action."Update Pulse Timings") -> ("error out"=w289:errorcluster)  [unwired: 8 in]
      }
      event "start sequence": Value Change {
        n111 = event-data() -> ("NewVal"=w294:bool)  [unwired: 1 in]
        n112 = case shown="True" w294 {
          tunnel: w298 -> [w304 w315]
          tunnel: w297 -> [w305 w314]
          tunnel: [w305 w312] -> w296
          tunnel: [w303 w306] -> w295
          frame False {
            n113 = Bundle By Name(cluster=cluster{"Abort?":bool} {"Abort?"=FALSE} ("General Flags Out"), "Abort?"=TRUE) -> (w299:cluster{"Abort?":bool})
            n114 = call "General Flags.vi"("General Flags In"=w299, "action"=General_Flags."Set Abort Flag" ("Action"), "error in"=w304) -> ("error out"=w303:errorcluster)  [unwired: 11 in, 1 out]
          }
          frame True {
            n115 = Enqueue Element(queue=w314, element=T19 {"data"=variant, "action"=enum."Start NMR DAQ"}, error in (no error)=w315) -> (queue out=w312:refnum<queue>, error out=w307:errorcluster)  [unwired: 1 in, 1 out]
            n116 = Bundle By Name(cluster=cluster{"Abort?":bool} {"Abort?"=FALSE} ("General Flags Out"), "Abort?"=FALSE) -> (w308:cluster{"Abort?":bool})
            n117 = call "General Flags.vi"("General Flags In"=w308, "action"=General_Flags."Set Abort Flag" ("Action"), "error in"=w307) -> ("error out"=w306:errorcluster)  [unwired: 11 in, 1 out]
          }
        }
      }
      event "start sequence  loop": Value Change {
        n118 = event-data() -> ("NewVal"=w316:bool)  [unwired: 1 in]
        n119 = case shown="True" w316 {
          tunnel: w319 -> [w326 w337]
          tunnel: w320 -> [w327 w336]
          tunnel: [w327 w334] -> w318
          tunnel: [w325 w328] -> w317
          frame False {
            n120 = Bundle By Name(cluster=cluster{"Abort?":bool} {"Abort?"=FALSE} ("General Flags Out"), "Abort?"=TRUE) -> (w321:cluster{"Abort?":bool})
            n121 = call "General Flags.vi"("General Flags In"=w321, "action"=General_Flags."Set Abort Flag" ("Action"), "error in"=w326) -> ("error out"=w325:errorcluster)  [unwired: 11 in, 1 out]
          }
          frame True {
            n122 = Enqueue Element(queue=w336, element=T19 {"data"=variant, "action"=enum."Start NMR DAQ Loop"}, error in (no error)=w337) -> (queue out=w334:refnum<queue>, error out=w329:errorcluster)  [unwired: 1 in, 1 out]
            n123 = Bundle By Name(cluster=cluster{"Abort?":bool} {"Abort?"=FALSE} ("General Flags Out"), "Abort?"=FALSE) -> (w330:cluster{"Abort?":bool})
            n124 = call "General Flags.vi"("General Flags In"=w330, "action"=General_Flags."Set Abort Flag" ("Action"), "error in"=w329) -> ("error out"=w328:errorcluster)  [unwired: 11 in, 1 out]
          }
        }
      }
      event Value Change {
        n125 = event-data() -> ("NewVal"=w344:T9)  [unwired: 1 in]
        n126 = Unbundle By Name(w344) -> ("Preliminary Settings.Nº of Echoes (ne)"=w345:u16, "Acquisition Settings.Number Samples"=w339:u16)
        n127 = Multiply(x=w345, y=w339) -> (x*y=w348:u16)
        n128 = Greater?(x=w348, y=u16 8000) -> (0:w346:bool)
        n129 = case shown="True" w346 {
          tunnel: w345 -> [_ w358]
          tunnel: [w356 w357] -> w343
          tunnel: w339 -> [w356 _]
          frame False {
          }
          frame True {
            n130 = Divide(x=u16 8000 ("y"), y=w358) -> (x/y=w357:ext)
          }
        }
        n131 = To Unsigned Word Integer(number=w343) -> (unsigned 16bit integer=w342:u16)
        n132 = Bundle By Name(cluster=w344, "Acquisition Settings.Number Samples"=w342) -> (w338:T9)
        n133 = property on="CPMG Pulse Sequence" class="Clust (strict)"(error in=w341, "Value"=w338) -> (error out=w340:errorcluster)  [unwired: 1 in, 1 out]
        n134 = call "Pulse Parameters.vi"("action"=Pulse_Parameters."Set CPMG Pulse Settings", "CPMG Pulse Sequence"=w338, "error in"=w340) -> ("error out"=w352:errorcluster)  [unwired: 5 in, 7 out]
        n135 = property on="Pulse Sequence Type" class="Enum (strict)"(error in=w352) -> (error out=w351:errorcluster, "Value"=w350:T3)  [unwired: 1 in, 1 out]
        n136 = call "User Interface Global.vi"("error in"=w351, "data1"=w350, "action"=User_Interface_Action."Update Pulse Timings") -> ("error out"=w349:errorcluster)  [unwired: 8 in]
      }
      event Value Change {
        n137 = event-data() -> ("NewVal"=w360:T13)  [unwired: 1 in]
        n138 = call "Pulse Parameters.vi"("T1 Pulse Sequence"=w360, "action"=Pulse_Parameters."Set T1 Pulse Settings", "error in"=w367) -> ("error out"=w363:errorcluster)  [unwired: 5 in, 7 out]
        n139 = property on="Pulse Sequence Type" class="Enum (strict)"(error in=w363) -> (error out=w362:errorcluster, "Value"=w361:T3)  [unwired: 1 in, 1 out]
        n140 = call "User Interface Global.vi"("error in"=w362, "data1"=w361, "action"=User_Interface_Action."Update Pulse Timings") -> ("error out"=w364:errorcluster)  [unwired: 8 in]
      }
      event Value Change {
        n141 = event-data() -> ("NewVal"=w382:bool)  [unwired: 1 in]
        n142 = property on="Hardware CTRL" class="Clust (strict)"(error in=w373) -> (error out=w372:errorcluster, "Value"=w371:T30)  [unwired: 1 in, 1 out]
        n143 = Not(x=w382) -> (.not. x?=w374:bool)
        n144 = property on="Start AQS" class="Bool (strict)"("Value"=w374) -> ()  [unwired: 2 in, 2 out]
        n145 = call "Hardware Parameters.vi"("action"=Hardware_Parameters."Set Hardware Settings", "error in"=w372, "Hardware Parameters"=w371) -> ("error out"=w376:errorcluster)  [unwired: 7 in, 1 out]
        n146 = Enqueue Element(queue=w378, element=T19 {"data"=variant, "action"=enum."Start AQS"}, error in (no error)=w376) -> (queue out=w377:refnum<queue>, error out=w370:errorcluster)  [unwired: 1 in, 1 out]
        n147 = call "User Interface Global.vi"("error in"=w370, "data1"="Start AQS", "action"=User_Interface_Action."Update Status Bar") -> ("error out"=w369:errorcluster)  [unwired: 8 in]
      }
      event Value Change {
        n148 = event-data() -> ("NewVal"=w395:bool)  [unwired: 1 in]
        n149 = property on="Hardware CTRL" class="Clust (strict)"(error in=w387) -> (error out=w386:errorcluster, "Value"=w385:T30)  [unwired: 1 in, 1 out]
        n150 = call "Hardware Parameters.vi"("action"=Hardware_Parameters."Set Hardware Settings", "error in"=w386, "Hardware Parameters"=w385) -> ("error out"=w389:errorcluster)  [unwired: 7 in, 1 out]
        n151 = Select(t="On", s=w395, f="Off") -> (s? t:f=w392:string)
        n152 = Enqueue Element(queue=w398, element=T19 {"data"=variant, "action"=enum."Set TX SW"}, error in (no error)=w389) -> (queue out=w397:refnum<queue>, error out=w384:errorcluster)  [unwired: 1 in, 1 out]
        n153 = Concatenate Strings("TX SW ", w392) -> (w390:string)
        n154 = call "User Interface Global.vi"("error in"=w384, "data1"=w390, "action"=User_Interface_Action."Update Status Bar") -> ("error out"=w383:errorcluster)  [unwired: 8 in]
      }
      event Value Change {
        n155 = event-data() -> ("NewVal"=w407:bool)  [unwired: 1 in]
        n156 = property on="Hardware CTRL" class="Clust (strict)"(error in=w404) -> (error out=w403:errorcluster, "Value"=w402:T30)  [unwired: 1 in, 1 out]
        n157 = call "Hardware Parameters.vi"("action"=Hardware_Parameters."Set Hardware Settings", "error in"=w403, "Hardware Parameters"=w402) -> ("error out"=w406:errorcluster)  [unwired: 7 in, 1 out]
        n158 = Select(t="On", s=w407, f="Off") -> (s? t:f=w410:string)
        n159 = Concatenate Strings("Rx SW ", w410) -> (w408:string)
        n160 = Enqueue Element(queue=w415, element=T19 {"data"=variant, "action"=enum."Set RX SW"}, error in (no error)=w406) -> (queue out=w414:refnum<queue>, error out=w401:errorcluster)  [unwired: 1 in, 1 out]
        n161 = call "User Interface Global.vi"("error in"=w401, "data1"=w408, "action"=User_Interface_Action."Update Status Bar") -> ("error out"=w400:errorcluster)  [unwired: 8 in]
      }
      event Value Change {
        n162 = event-data() -> ("NewVal"=w425:bool)  [unwired: 1 in]
        n163 = Not(x=w425) -> (.not. x?=w422:bool)
        n164 = property on="Hardware CTRL" class="Clust (strict)"(error in=w421) -> (error out=w420:errorcluster, "Value"=w419:T30)  [unwired: 1 in, 1 out]
        n165 = property on="Send Pulse" class="Bool (strict)"("Value"=w422) -> ()  [unwired: 2 in, 2 out]
        n166 = call "Hardware Parameters.vi"("action"=Hardware_Parameters."Set Hardware Settings", "error in"=w420, "Hardware Parameters"=w419) -> ("error out"=w424:errorcluster)  [unwired: 7 in, 1 out]
        n167 = Enqueue Element(queue=w429, element=T19 {"data"=variant, "action"=enum."Send Pulse"}, error in (no error)=w424) -> (queue out=w428:refnum<queue>, error out=w418:errorcluster)  [unwired: 1 in, 1 out]
        n168 = call "User Interface Global.vi"("error in"=w418, "data1"="Pulse Sent", "action"=User_Interface_Action."Update Status Bar") -> ("error out"=w417:errorcluster)  [unwired: 8 in]
      }
      event Value Change {
        n169 = event-data() -> ()  [unwired: 1 in, 1 out]
        n170 = property on="Hardware CTRL" class="Clust (strict)"(error in=w435) -> (error out=w434:errorcluster, "Value"=w433:T30)  [unwired: 1 in, 1 out]
        n171 = call "Hardware Parameters.vi"("action"=Hardware_Parameters."Set Hardware Settings", "error in"=w434, "Hardware Parameters"=w433) -> ("error out"=w437:errorcluster)  [unwired: 7 in, 1 out]
        n172 = Enqueue Element(queue=w441, element=T19 {"data"=variant, "action"=enum."Set CutOff Freq1"}, error in (no error)=w437) -> (queue out=w440:refnum<queue>, error out=w432:errorcluster)  [unwired: 1 in, 1 out]
        n173 = call "User Interface Global.vi"("error in"=w432, "data1"="CutOff Freq1 Set", "action"=User_Interface_Action."Update Status Bar") -> ("error out"=w431:errorcluster)  [unwired: 8 in]
      }
      event Value Change {
        n174 = event-data() -> ()  [unwired: 1 in, 1 out]
        n175 = property on="Hardware CTRL" class="Clust (strict)"(error in=w447) -> (error out=w446:errorcluster, "Value"=w445:T30)  [unwired: 1 in, 1 out]
        n176 = call "Hardware Parameters.vi"("action"=Hardware_Parameters."Set Hardware Settings", "error in"=w446, "Hardware Parameters"=w445) -> ("error out"=w449:errorcluster)  [unwired: 7 in, 1 out]
        n177 = Enqueue Element(queue=w453, element=T19 {"data"=variant, "action"=enum."Set CutOff Freq2"}, error in (no error)=w449) -> (queue out=w452:refnum<queue>, error out=w444:errorcluster)  [unwired: 1 in, 1 out]
        n178 = call "User Interface Global.vi"("error in"=w444, "data1"="CutOff Freq2 Set", "action"=User_Interface_Action."Update Status Bar") -> ("error out"=w443:errorcluster)  [unwired: 8 in]
      }
      event Value Change {
        n179 = event-data() -> ("NewVal"=w463:bool)  [unwired: 1 in]
        n180 = property on="Hardware CTRL" class="Clust (strict)"(error in=w459) -> (error out=w458:errorcluster, "Value"=w457:T30)  [unwired: 1 in, 1 out]
        n181 = Not(x=w463) -> (.not. x?=w460:bool)
        n182 = property on="Reset DDS" class="Bool (strict)"("Value"=w460) -> ()  [unwired: 2 in, 2 out]
        n183 = call "Hardware Parameters.vi"("action"=Hardware_Parameters."Set Hardware Settings", "error in"=w458, "Hardware Parameters"=w457) -> ("error out"=w462:errorcluster)  [unwired: 7 in, 1 out]
        n184 = Enqueue Element(queue=w467, element=T19 {"data"=variant, "action"=enum."Reset DDS"}, error in (no error)=w462) -> (queue out=w466:refnum<queue>, error out=w456:errorcluster)  [unwired: 1 in, 1 out]
        n185 = call "User Interface Global.vi"("error in"=w456, "data1"="Reset DDS", "action"=User_Interface_Action."Update Status Bar") -> ("error out"=w455:errorcluster)  [unwired: 8 in]
      }
      event Value Change {
        n186 = event-data() -> ("NewVal"=w477:bool)  [unwired: 1 in]
        n187 = property on="Hardware CTRL" class="Clust (strict)"(error in=w473) -> (error out=w472:errorcluster, "Value"=w471:T30)  [unwired: 1 in, 1 out]
        n188 = Not(x=w477) -> (.not. x?=w474:bool)
        n189 = property on="Set DDS" class="Bool (strict)"("Value"=w474) -> ()  [unwired: 2 in, 2 out]
        n190 = call "Hardware Parameters.vi"("action"=Hardware_Parameters."Set Hardware Settings", "error in"=w472, "Hardware Parameters"=w471) -> ("error out"=w475:errorcluster)  [unwired: 7 in, 1 out]
        n191 = Enqueue Element(queue=w481, element=T19 {"data"=variant, "action"=enum."Set DDS"}, error in (no error)=w475) -> (queue out=w480:refnum<queue>, error out=w470:errorcluster)  [unwired: 1 in, 1 out]
        n192 = call "User Interface Global.vi"("error in"=w470, "data1"="Set DDS", "action"=User_Interface_Action."Update Status Bar") -> ("error out"=w469:errorcluster)  [unwired: 8 in]
      }
      event Value Change {
        n193 = event-data() -> ()  [unwired: 1 in, 1 out]
        n194 = property on="Hardware CTRL" class="Clust (strict)"(error in=w487) -> (error out=w486:errorcluster, "Value"=w485:T30)  [unwired: 1 in, 1 out]
        n195 = call "Hardware Parameters.vi"("action"=Hardware_Parameters."Set Hardware Settings", "error in"=w486, "Hardware Parameters"=w485) -> ("error out"=w489:errorcluster)  [unwired: 7 in, 1 out]
        n196 = Enqueue Element(queue=w493, element=T19 {"data"=variant, "action"=enum."Set Gain1"}, error in (no error)=w489) -> (queue out=w492:refnum<queue>, error out=w484:errorcluster)  [unwired: 1 in, 1 out]
        n197 = call "User Interface Global.vi"("error in"=w484, "data1"="Set GAin1", "action"=User_Interface_Action."Update Status Bar") -> ("error out"=w483:errorcluster)  [unwired: 8 in]
      }
      event Value Change {
        n198 = event-data() -> ()  [unwired: 1 in, 1 out]
        n199 = property on="Hardware CTRL" class="Clust (strict)"(error in=w499) -> (error out=w498:errorcluster, "Value"=w497:T30)  [unwired: 1 in, 1 out]
        n200 = call "Hardware Parameters.vi"("action"=Hardware_Parameters."Set Hardware Settings", "error in"=w498, "Hardware Parameters"=w497) -> ("error out"=w501:errorcluster)  [unwired: 7 in, 1 out]
        n201 = Enqueue Element(queue=w505, element=T19 {"data"=variant, "action"=enum."Set Gain2"}, error in (no error)=w501) -> (queue out=w502:refnum<queue>, error out=w496:errorcluster)  [unwired: 1 in, 1 out]
        n202 = call "User Interface Global.vi"("error in"=w496, "data1"="Set Gain2", "action"=User_Interface_Action."Update Status Bar") -> ("error out"=w495:errorcluster)  [unwired: 8 in]
      }
      event Value Change {
        n203 = event-data() -> ("NewVal"=w508:T3)  [unwired: 1 in]
        n204 = call "User Interface Global.vi"("error in"=w510, "data1"=w508, "action"=User_Interface_Action."Set Pulse Sequence Type") -> ("error out"=w507:errorcluster)  [unwired: 8 in]
      }
    }
    n205 = call "Error Module.vi"("error in"=w255) -> ("error out"=w254:errorcluster)  [unwired: 9 in, 1 out]
  }
  n206 = while {
    shift-right: [w518] -> w14
    shift-left: w5 -> [w524]
    shift-right: [w515] -> w16
    shift-left: w20 -> [w525]
    shift-right: [w512] -> _
    shift-left: w1 -> [w513]
    stop <- w517 stop-if-true
    n207 = Dequeue Element(queue=w524, error in (no error)=w525) -> (queue out=w519:refnum<queue>, element=w523:T17, error out=w521:errorcluster)  [unwired: 1 in, 1 out]
    n208 = Unbundle By Name(w523) -> ("action"=w522:T18, "data1"=w520:variant, "data2"=w514:variant)
    n209 = case shown="\"Initialize\", Default" w522 {
      tunnel: w521 -> [w531 w543 w552 w572 w574 w586 w602 w616 w668 w675 w683 w691 w699 w707 w711]
      tunnel: w520 -> [_ w542 w553 w571 _ w587 w601 w615 w667 w674 w681 w689 w697 w705 _]
      tunnel: w519 -> [w533 w544 w555 w570 w575 w588 w593 w610 w664 w676 w678 w685 w693 w701 w710]
      tunnel: [w533 w544 w555 w570 w575 w588 w593 w610 w664 w676 w678 w685 w693 w701 w710] -> w518
      tunnel: [w527 w539 w547 w569 w574 w577 w594 w611 w665 w671 w679 w687 w694 w703 w711] -> w516
      tunnel: [_ _ _ _ _ _ _ _ _ _ _ _ _ _ TRUE] -> w517
      tunnel: w514 -> [_ w536 w549 _ _ _ _ _ _ _ _ _ _ _ _]
      tunnel: w513 -> [w532 w540 w551 w556 w573 w578 w589 w609 w663 w670 w677 w684 w692 w700 w708]
      tunnel: [w532 w540 w551 w556 w573 w578 w589 w609 w663 w670 w677 w684 w692 w700 w708] -> w512
      frame "Initialize", Default {
        w526 = FALSE ("Value")
        n210 = property on="Start AQS" class="Bool (strict)"(error in=w531, "Value"=w526) -> (error out=w530:errorcluster)  [unwired: 1 in, 1 out]
        n211 = property on="Send Pulse" class="Bool (strict)"(error in=w530, "Value"=w526) -> (error out=w529:errorcluster)  [unwired: 1 in, 1 out]
        n212 = property on="Reset DDS" class="Bool (strict)"(error in=w529, "Value"=w526) -> (error out=w528:errorcluster)  [unwired: 1 in, 1 out]
        n213 = property on="Set DDS" class="Bool (strict)"(error in=w528, "Value"=w526) -> (error out=w527:errorcluster)  [unwired: 1 in, 1 out]
      }
      frame "Update Real Channel" {
        n214 = Variant To Data(error in=w543, type=cluster{"magnitude":dbl[], dbl[]} {"magnitude"=array[2501 elements], array[2500 elements]} ("Real"), Variant=w542) -> (data=→"Real (Freq Domain)":cluster{"magnitude":dbl[], dbl[]}, error out=w538:errorcluster)
        n215 = Variant To Data(error in=w538, type=cluster{"magnitude":dbl[], dbl[]} {"magnitude"=[0.0, 678000.1166160201], [19.552127862926234]} ("FFT Real 2"), Variant=w536) -> (data=→"Real (time Domain)":cluster{"magnitude":dbl[], dbl[]}, error out=w539:errorcluster)
      }
      frame "Update Imag Channel" {
        n216 = Variant To Data(error in=w552, type=cluster{"magnitude":dbl[], dbl[]} {"magnitude"=array[2501 elements], array[2500 elements]} ("Real"), Variant=w553) -> (data=→"Imag (Freq Domain)":cluster{"magnitude":dbl[], dbl[]}, error out=w550:errorcluster)
        n217 = Variant To Data(error in=w550, type=cluster{"magnitude":dbl[], dbl[]} {"magnitude"=array[2501 elements], array[2500 elements]} ("Real"), Variant=w549) -> (data=→"Imag (time Domain)":cluster{"magnitude":dbl[], dbl[]}, error out=w547:errorcluster)
      }
      frame "Update Re/Im channel @ Hardware Ctrl" {
        n218 = Variant To Data(error in=w572, type=cluster{"magnitude":dbl[], dbl[]}[] [] ("appended array"), Variant=w571) -> (data=w559:cluster{"magnitude":dbl[], dbl[]}[], error out=w569:errorcluster)
        n219 = Index Array(array=w559, index #1=0 ("index"), index #2=2 ("index")) -> (element #1=w564:cluster{"magnitude":dbl[], dbl[]}, element #2=w565:cluster{"magnitude":dbl[], dbl[]})
        n220 = Index Array(array=w559, index #1=1 ("index"), index #2=3 ("index")) -> (element #1=w563:cluster{"magnitude":dbl[], dbl[]}, element #2=w562:cluster{"magnitude":dbl[], dbl[]})
        n221 = Build Array(w564, w565) -> (→"FFT Graph":cluster{"magnitude":dbl[], dbl[]}[])
        n222 = Build Array(w563, w562) -> (→"Time Graph":cluster{"magnitude":dbl[], dbl[]}[])
      }
      frame "Visibility Front Panel Controls" {
      }
      frame "Report Custom Errors" {
        w576 = T32 2 items=["no dialog", "OK message", "continue or stop message", "OK message + warnings", "continue/stop + warnings"] ("type of dialog (OK msg:1)")
        n223 = Variant To Data(error in=w586, type=0, Variant=w587) -> (data=w584:i32, error out=w583:errorcluster)
        n224 = Unbundle By Name(T31 {"[user-defined codes]"=[5000, 5001, 5002, 5003, 5004, 5005, 5006, 5007, 5008, 5009, 5010, 5011, 5012, 6000, 0, 0, 0, 0, 0, 0, 0, 5000], "[user-defined descriptions]"=["Set DDS Error - Restart Program and Try again", "Send DDS Pulse Error - Restart Program and Try again", "Reset DDS Error - Restart Program and Try again", "Tx Sw Control Error - Restart Program and Try again", "Rx Sw Control Error - Restart Program and Try again", "Set CutOff Freq1 Error - Restart Program and Try again", "Set Gain1 Error - Restart Program and Try again", "Set CutOff Freq2 Error - Restart Program and Try again", "Set Gain2 Error  - Restart Program and Try again", "Hardware AQS test Error - Restart Program and Try again", "", "", "", "Device Not present - Restart Program and Try again"]} ("Custom Errors")) -> ("[user-defined codes]"=w581:i32[], "[user-defined descriptions]"=w582:string[])
        n225 = call <vilib>:"General Error Handler.vi"("[error code] (0)"=w584, "[user-defined codes]"=w581, "[user-defined descriptions]"=w582, "[error source] (\" \")"="NMR Program" ("[error source] (\" \")"), "type of dialog (OK msg:1)"=w576, "error in (no error)"=w583) -> ("error out"=w577:errorcluster)  [unwired: 5 in, 4 out]
      }
      frame "Set Pulse Sequence Type" {
        n226 = Variant To Data(error in=w602, type=0, Variant=w601) -> (data=w590:i32, error out=w592:errorcluster)
        n227 = property on="Pulse Sequence Type" class="Enum (strict)"(error in=w592, "Value"=w590) -> (error out=w591:errorcluster)  [unwired: 1 in, 1 out]
        n228 = case shown="0, Default" w590 {
          tunnel: [TRUE w605 w608] -> w599
          tunnel: [w603 w605 TRUE] -> w598
          tunnel: [w603 TRUE w608] -> w597
          frame 0, Default {
            w603 = FALSE
          }
          frame 1 {
            w605 = FALSE
          }
          frame 2 {
            w608 = FALSE
          }
        }
        n229 = property on="T1 Pulse Sequence" class="Clust (strict)"(error in=w591, "Visible"=w598) -> (error out=w596:errorcluster)  [unwired: 1 in, 1 out]
        n230 = property on="CPMG Pulse Sequence" class="Clust (strict)"(error in=w596, "Visible"=w597) -> (error out=w595:errorcluster)  [unwired: 1 in, 1 out]
        n231 = property on="90 Degree Pulse Sequence" class="Clust (strict)"(error in=w595, "Visible"=w599) -> (error out=w594:errorcluster)  [unwired: 1 in, 1 out]
      }
      frame "Update Pulse Timings" {
        n232 = Variant To Data(error in=w616, type=NMR_Pulse_Sequence_Type."90 Degree Sequence" ("Pulse Sequence Type"), Variant=w615) -> (data=w613:T3, error out=w614:errorcluster)
        n233 = case shown="\"T1 Pulse Sequence\"" w613 {
          tunnel: w614 -> [w627 w645 w661]
          tunnel: [w620 w632 w653] -> w611
          frame "90 Degree Sequence", Default {
            n234 = call "Pulse Parameters.vi"("action"=Pulse_Parameters."Get 90 Degree Settings", "error in"=w627) -> ("Set Time 90 Degree Pulse"=w626:T33, "error out"=w619:errorcluster)  [unwired: 6 in, 6 out]
            n235 = Unbundle By Name(w626) -> ("D1 Real Time"=w618:ext, "D2 Real Time"=w623:ext, "P1 Real Time"=w622:ext, "AQS Real Time"=w621:ext)
            n236 = property on="Delay d1" class="DigNum (strict)"(error in=w619, "Value"=w618) -> (error out=w617:errorcluster)  [unwired: 1 in, 1 out]
            n237 = property on="Delay d2" class="DigNum (strict)"(error in=w617, "Value"=w623) -> (error out=w625:errorcluster)  [unwired: 1 in, 1 out]
            n238 = property on="Duration Signal P1" class="DigNum (strict)"(error in=w625, "Value"=w622) -> (error out=w624:errorcluster)  [unwired: 1 in, 1 out]
            n239 = property on="Time Between Points" class="DigNum (strict)"(error in=w624, "Value"=w621) -> (error out=w620:errorcluster)  [unwired: 1 in, 1 out]
          }
          frame "CPMG Pulse Sequence" {
            n240 = call "Pulse Parameters.vi"("action"=Pulse_Parameters."Get CPMG Settings", "error in"=w645) -> ("CPMG Set Times"=w644:T34, "error out"=w643:errorcluster)  [unwired: 6 in, 6 out]
            n241 = Unbundle By Name(w644) -> ("Real Time d1"=w642:ext, "Real Time d2"=w638:ext, "Real Time d3"=w637:ext, "Real Time d4"=w636:ext, "Real Time P1"=w631:ext, "Real Time P2"=w630:ext, "Real Time AQS"=w629:ext)
            n242 = property on="Delay d1" class="DigNum (strict)"(error in=w643, "Value"=w642) -> (error out=w641:errorcluster)  [unwired: 1 in, 1 out]
            n243 = property on="Delay d2" class="DigNum (strict)"(error in=w641, "Value"=w638) -> (error out=w640:errorcluster)  [unwired: 1 in, 1 out]
            n244 = property on="Delay d3" class="DigNum (strict)"(error in=w640, "Value"=w637) -> (error out=w639:errorcluster)  [unwired: 1 in, 1 out]
            n245 = property on="Delay d4" class="DigNum (strict)"(error in=w639, "Value"=w636) -> (error out=w635:errorcluster)  [unwired: 1 in, 1 out]
            n246 = property on="Duration Signal P1" class="DigNum (strict)"(error in=w635, "Value"=w631) -> (error out=w634:errorcluster)  [unwired: 1 in, 1 out]
            n247 = property on="Duration Signal P2" class="DigNum (strict)"(error in=w634, "Value"=w630) -> (error out=w633:errorcluster)  [unwired: 1 in, 1 out]
            n248 = property on="Time Between Points" class="DigNum (strict)"(error in=w633, "Value"=w629) -> (error out=w632:errorcluster)  [unwired: 1 in, 1 out]
          }
          frame "T1 Pulse Sequence" {
            n249 = call "Pulse Parameters.vi"("action"=Pulse_Parameters."Get T1 Settings", "error in"=w661) -> ("T1 set times"=w660:T35, "error out"=w658:errorcluster)  [unwired: 6 in, 6 out]
            n250 = Unbundle By Name(w660) -> ("Real Time d1"=w657:ext, "Real Time d2"=w656:ext, "Real Time d30"=w654:ext, "Real Time P1"=w651:ext, "Real Time P2"=w650:ext, "Real Time AQS"=w652:ext)
            n251 = property on="Delay d1" class="DigNum (strict)"(error in=w658, "Value"=w657) -> (error out=w659:errorcluster)  [unwired: 1 in, 1 out]
            n252 = property on="Delay d2" class="DigNum (strict)"(error in=w659, "Value"=w656) -> (error out=w655:errorcluster)  [unwired: 1 in, 1 out]
            n253 = property on="Delay d30" class="DigNum (strict)"(error in=w655, "Value"=w654) -> (error out=w648:errorcluster)  [unwired: 1 in, 1 out]
            n254 = property on="Duration Signal P1" class="DigNum (strict)"(error in=w648, "Value"=w651) -> (error out=w649:errorcluster)  [unwired: 1 in, 1 out]
            n255 = property on="Duration Signal P2" class="DigNum (strict)"(error in=w649, "Value"=w650) -> (error out=w647:errorcluster)  [unwired: 1 in, 1 out]
            n256 = property on="Time Between Points" class="DigNum (strict)"(error in=w647, "Value"=w652) -> (error out=w653:errorcluster)  [unwired: 1 in, 1 out]
          }
        }
      }
      frame "Update Transfer Time" {
        n257 = Variant To Data(error in=w668, type=u32 0 ("Sequence Progress"), Variant=w667) -> (data=→"Transfer Time (ms)":u32, error out=w665:errorcluster)
      }
      frame "Update Status Bar" {
        n258 = Variant To Data(error in=w675, type="", Variant=w674) -> (data=→"Status Bar":string, error out=w671:errorcluster)
      }
      frame "Set Sequence Progress" {
        n259 = Variant To Data(error in=w683, type=u32 0 ("Sequence Progress"), Variant=w681) -> (data=→"Sequence Progress":u32, error out=w679:errorcluster)
      }
      frame "Set 90 Degree Pulse Sequence Params" {
        n260 = Variant To Data(error in=w691, type=T25 {"Delay Settings"={"Delay d1"=83.9713885729285, "Delay d2"=94.03351124332838, "d1 Unit"=0, "d2 Unit"=0}, "Preliminary Settings"={"Nº of Scans (ns)"=22, "Pulse Frequency"=10000000.0}, "Pulse Settings"={"Duration Signal P1"=20.97375098433809, "Power Level"=1023, "Phase"=90, "P1 Units"=0}, "Acquisition Settings"={"Number Samples"=2000, "Time Between Points"=0.737463, "Unit"=0}}, Variant=w689) -> (data=w686:T25, error out=w688:errorcluster)
        n261 = property on="90 Degree Pulse Sequence" class="Clust (strict)"(error in=w688, "Value"=w686) -> (error out=w687:errorcluster)  [unwired: 1 in, 1 out]
      }
      frame "Set CMPG Pulse Sequence Parms" {
        n262 = Variant To Data(error in=w699, type=T26 {"Acquisition Settings"={"Number Samples"=2000, "Time Between Points"=0.737463, "Unit"=0}, "Delay Settings"={"Delay d1"=10.99912503281127, "Delay d2"=8.024236591127833, "d1 Unit"=0, "d2 Unit"=0, "Delay d3"=8.986700498731297, "d3 Unit"=0, "Delay d4"=27.011024586578003, "d4 Unit"=0}, "Preliminary Settings"={"Nº of Scans (ns)"=3, "Pulse Frequency"=10000000.0, "Nº of Echoes (ne)"=3}, "Pulse Settings"={"Duration Signal P1"=36.02318663050136, "Power Level P1"=1021, "Phase P1"=90, "P1 Unit"=0, "Duration Signal P2"=8.986700498731297, "Power Level P2"=1023, "Phase P2"=90, "P2 Unit"=0}}, Variant=w697) -> (data=w695:T26, error out=w696:errorcluster)
        n263 = property on="CPMG Pulse Sequence" class="Clust (strict)"(error in=w696, "Value"=w695) -> (error out=w694:errorcluster)  [unwired: 1 in, 1 out]
      }
      frame "Set T1 Pulse Sequence Params" {
        n264 = Variant To Data(error in=w707, type=T27 {"Preliminary Settings"={"Nº of Scans (ns)"=1, "Pulse Frequency"=11000000.0, "Nº of Vd"=2}, "Pulse Settings"={"Duration Signal P2"=20.01128707673462, "Power Level P2"=1023, "Phase P2"=90, "P2 Unit"=0, "Duration Signal P1"=20.01128707673462, "Power Level P1"=1023, "Phase P1"=90, "P1 Unit"=0}, "Acquisition Settings"={"Number Samples"=2000, "Time Between Points"=11.960617384240454, "Unit"=0}, "Delay Settings"={"Delay d1"=32.960801469944876, "Delay d2"=169.0181993175256, "d1 Unit"=0, "d2 Unit"=0, "Delay d30"=87.03377373348499, "d30 Unit"=0, "Vd Unit"=0, "Vd Values"="0"}}, Variant=w705) -> (data=w702:T27, error out=w704:errorcluster)
        n265 = property on="T1 Pulse Sequence" class="Clust (strict)"(error in=w704, "Value"=w702) -> (error out=w703:errorcluster)  [unwired: 1 in, 1 out]
      }
      frame "Stop" {
      }
    }
    n266 = call "Error Module.vi"("error in"=w516) -> ("error out"=w515:errorcluster)  [unwired: 9 in, 1 out]
  }
  n267 = Merge Errors(w18, w17, w16) -> (w13:errorcluster)
  n268 = Release Queue(queue=w15, error in (no error)=w13) -> (error out=w12:errorcluster)  [unwired: 1 in, 2 out]
  n269 = Release Queue(queue=w14, error in (no error)=w12) -> (error out=w11:errorcluster)  [unwired: 1 in, 2 out]
  n270 = Unregister For Events(event registration refnum=w26, error in=w11) -> (error out=w10:errorcluster)
  n271 = Destroy User Event(user event=w7, error in=w10) -> (error out=w2:errorcluster)
  n272 = call <vilib>:"Simple Error Handler.vi"("error in (no error)"=w2) -> ("error out"=w9:errorcluster)  [unwired: 4 in, 4 out]
  n273 = disable-structure shown="DEPLOY==TRUE" {
    disable-tunnel: w9 -> [_ _]
    frame condition #0 {
      n274 = Quit LabVIEW() -> ()  [unwired: 1 in]
    }
    frame condition #1 (active) {
    }
  }
